vi "Interpret Driver Controls.vi"() -> ()   [LabVIEW 2018]
uses:
  <vilib>/Rock Robotics/WPI/DriverStation/WPI_DriverStationDerivedRobotMode.ctl
  Robot Global Data.vi
  SubSystems/Controllers/Driver Controller/Driver Controller Global.vi
  SubSystems/Drive Train/Drive Train Global.vi
  SubSystems/Lift/Lift Global.vi
  <vilib>/addons/control/pid/pid.llb/PID (DBL).vi
  SubSystems/Controllers/Manipulator Controlller/Manipulator Controller Global.vi
  SubSystems/HAB Climber/HAB Climber Global.vi
  SubSystems/Hatch Panel Intake/Hatch Panel Intake Global.vi
  SubSystems/Cargo Intake/Cargo Intake Global.vi
  <vilib>/addons/control/pid/NI_PID_pid.lvlib
panel:
  in  "Last Move Deadband":u32=500
  in  "Last Time Auto":u32=1171826
  in  "Camera Tracking":T1={"proportional gain (Kc)"=0.06, "integral time (Ti, min)"=0.0, "derivative time (Td, min)"=0.0}
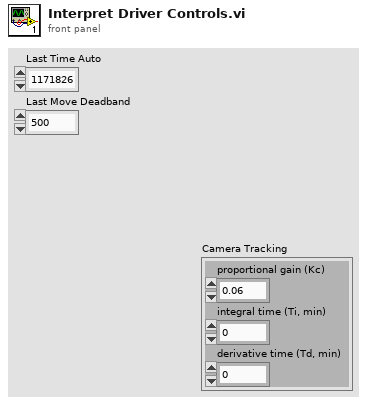
[diagram p1: front panel]
types:
  T1 = cluster{"proportional gain (Kc)":dbl, "integral time (Ti, min)":dbl, "derivative time (Td, min)":dbl}
  T2 = enum16{"Manual", "Hatch Panel Zone 1", "Hatch Panel Zone 2", "Hatch Panel Zone 3", "Cargo Zone 1", "Cargo Zone 2", "Cargo Zone 3", "Cargo Ship Zone"}
  T3 = cluster{"Rollover":dbl, "Yaw":dbl, "Cont Yaw":dbl}
  T4 = typedef "WPI_DriverStationDerivedRobotMode.ctl" = enum16{"Init", "Execute", "Stop"}
  T5 = enum16{"Hatch Panel Zone 1", "Hatch Panel Zone 2", "Hatch Panel Zone 3", "Cargo Zone 1", "Cargo Zone 2", "Cargo Zone 3", "Cargo Ship Zone"}
  T6 = cluster{"offsetAngle H":dbl, "offsetAngle V":dbl, "area":dbl, "skew":dbl, "validTarget":dbl, "latency":dbl}
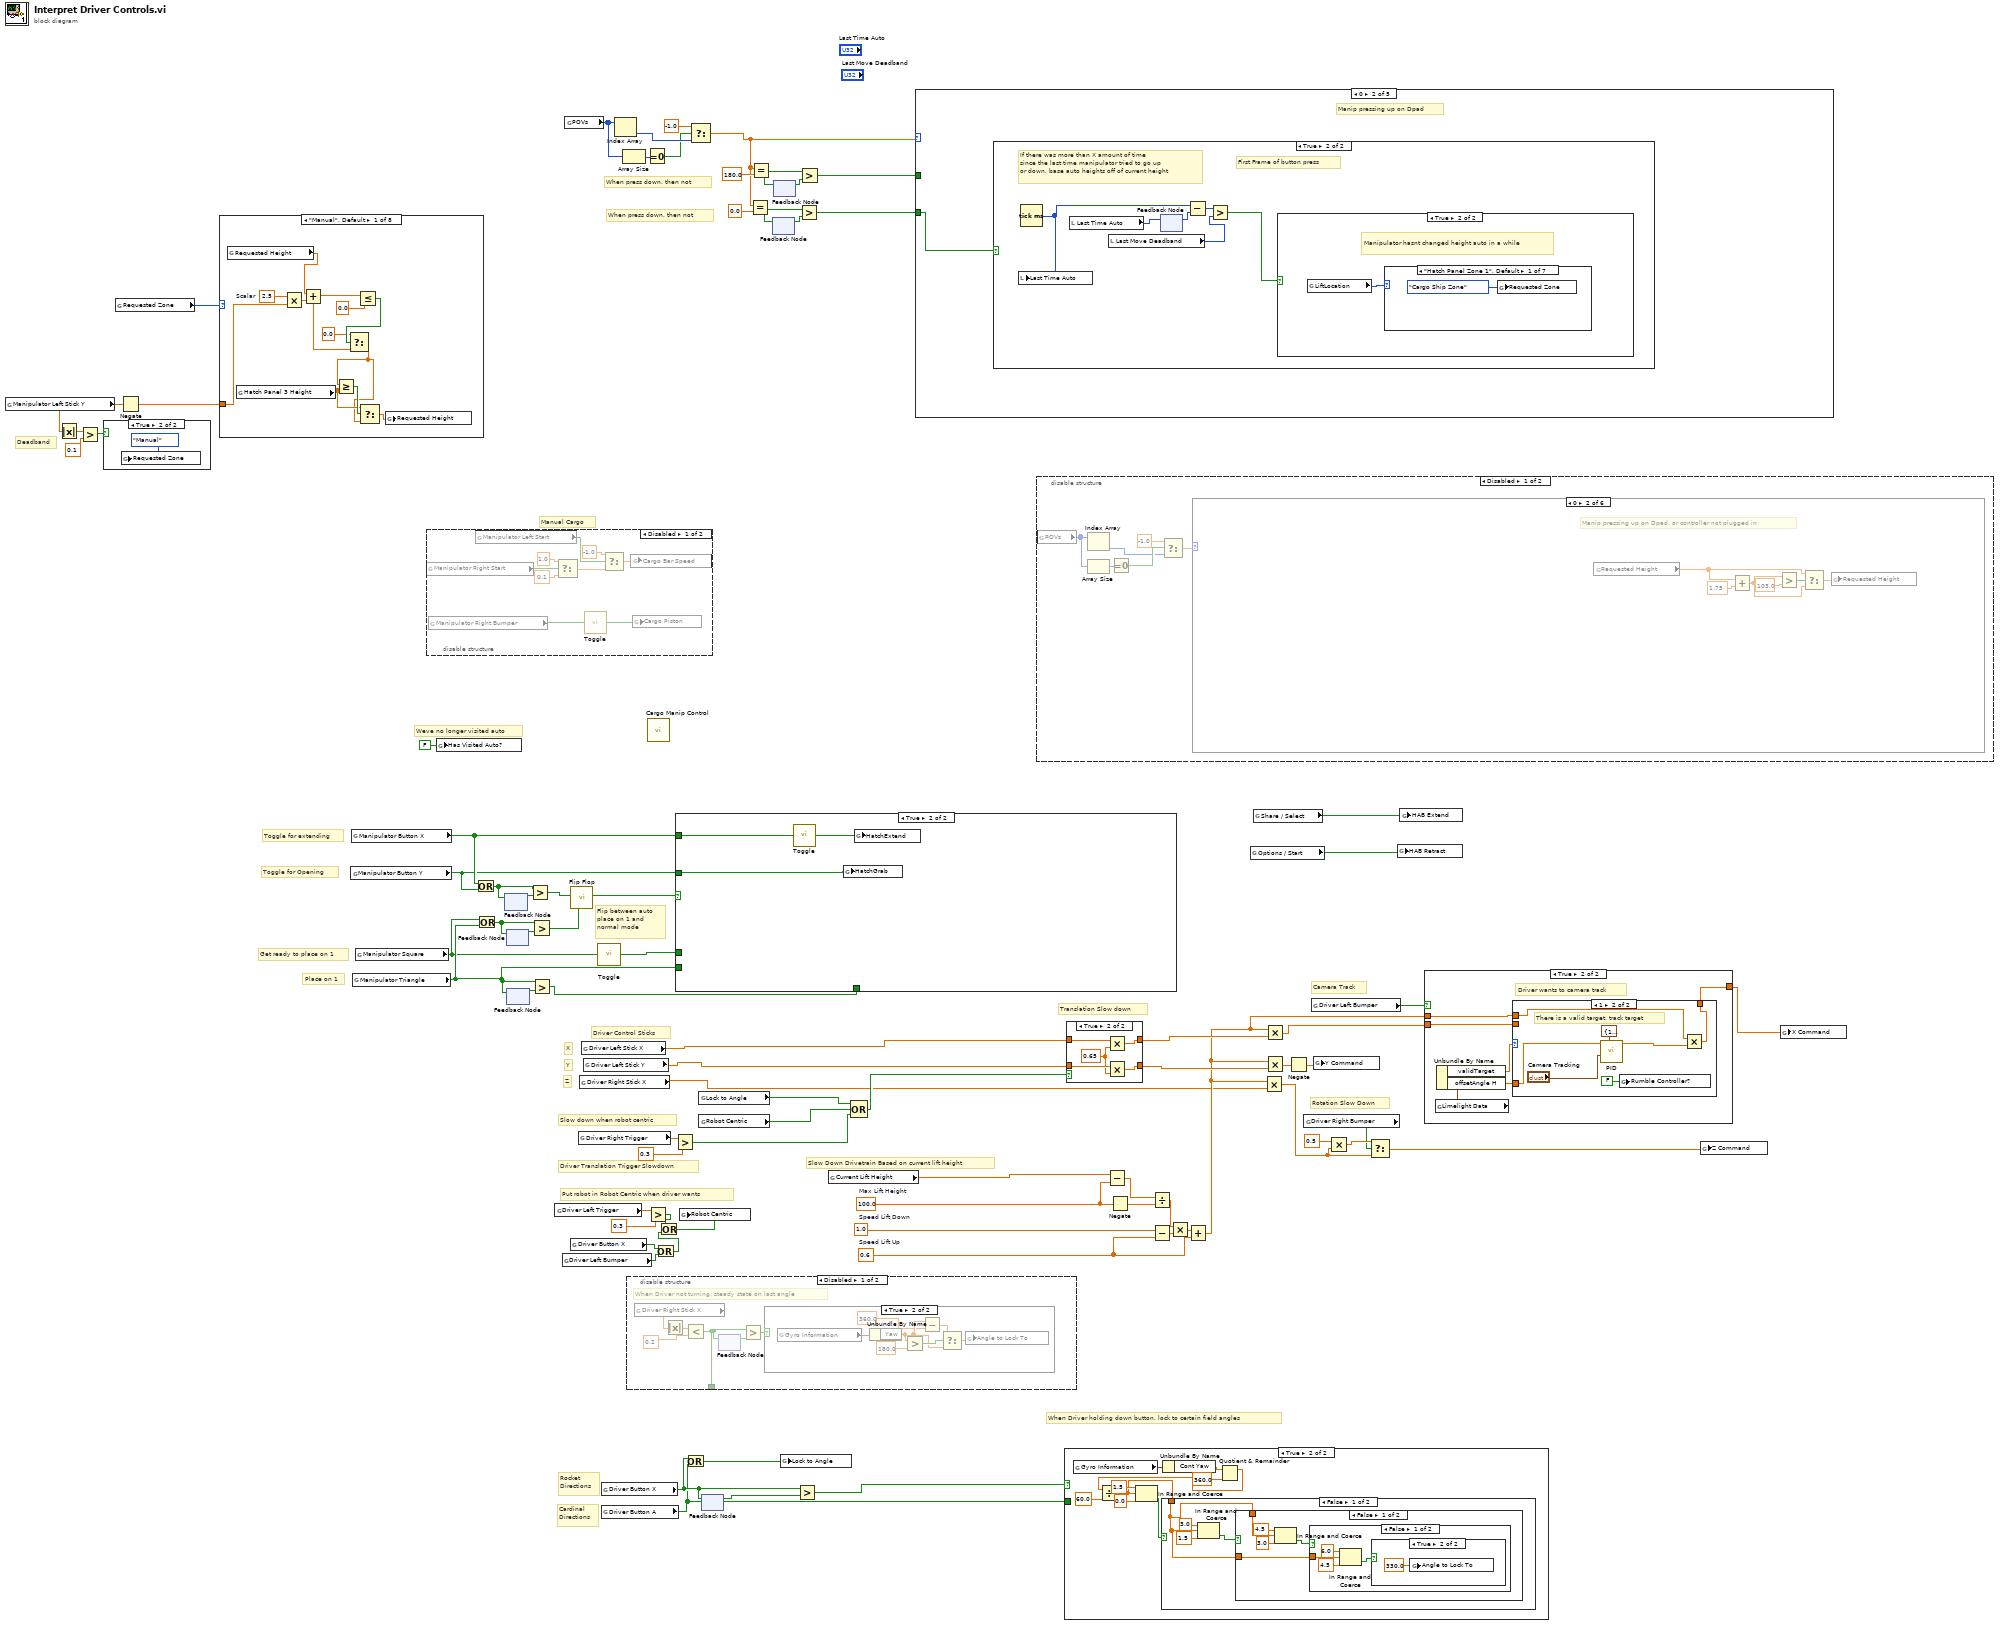
[diagram p0: block diagram]
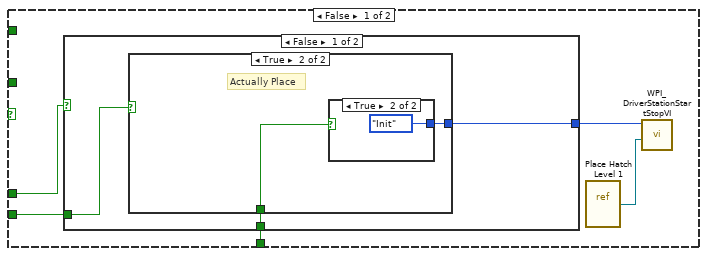
[diagram p2: hidden frame]
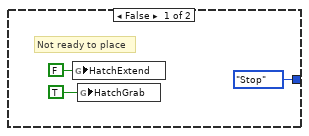
[diagram p3: hidden frame]
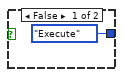
[diagram p4: hidden frame]
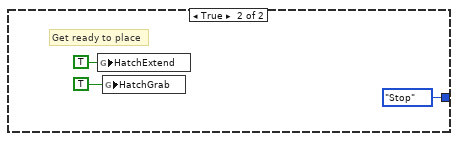
[diagram p5: hidden frame]
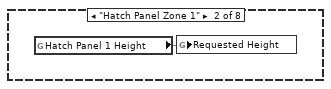
[diagram p7: hidden frame]
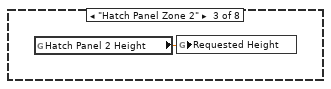
[diagram p8: hidden frame]
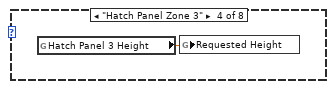
[diagram p9: hidden frame]
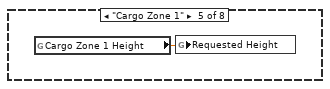
[diagram p10: hidden frame]
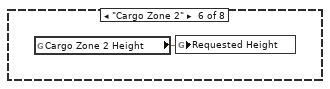
[diagram p11: hidden frame]
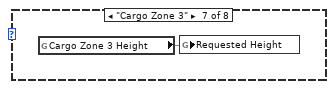
[diagram p12: hidden frame]
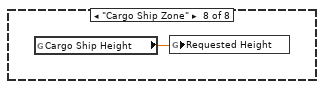
[diagram p13: hidden frame]
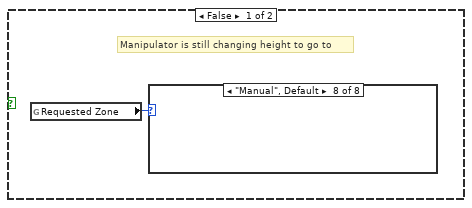
[diagram p16: hidden frame]
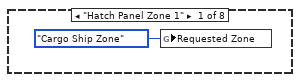
[diagram p17: hidden frame]
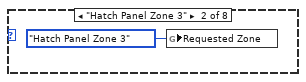
[diagram p18: hidden frame]
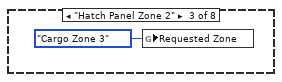
[diagram p19: hidden frame]
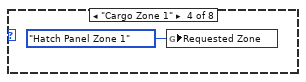
[diagram p20: hidden frame]
diagram:
  w61 = 0.6  # Speed Lift Up
  w65 = 1.0  # Speed Lift Down
  w59 = 100.0  # Max Lift Height
  # "Toggle for Opening"
  # "Toggle for extending"
  # "Place on 1"
  # "Get ready to place on 1"
  # "Flip between auto\nplace on 1 and \nnormal mode"
  # "When press down, then not"
  # "When press down, then not"
  # "Deadband"
  # "Manual Cargo"
  # "Weve no longer visited auto"
  # "Camera Track"
  # "Rotation Slow Down"
  # "Rocket\nDirections"
  # "Cardinal\nDirections"
  # "When Driver holding down button, lock to certain field angles"
  # "Slow Down Drivetrain Based on current lift height"
  # "Put robot in Robot Centric when driver wants"
  # "Slow down when robot centric"
  # "Driver Translation Trigger Slowdown"
  # "Translation Slow down"
  # "Z"
  # "Y"
  # "X"
  # "Driver Control Sticks"
  n1 = global read "Manipulator Controller Global.vi" "Manipulator Left Stick Y"() -> (w30:dbl)
  n2 = Absolute Value(x=w30) -> (abs(x)=w33:dbl)
  n3 = Greater?(x=w33, y=0.1) -> (0:w31:bool)
  n4 = case shown="True" w31 {
    frame False {
    }
    frame True {
      n5 = global write "Lift Global.vi" "Requested Zone"(T2."Manual" ("Requested Zone")) -> ()
    }
  }
  n6 = global read "Lift Global.vi" "Requested Zone"() -> (w34:T2)
  n7 = Negate(x=w30) -> (-x=w29:dbl)
  n8 = case shown="\"Manual\", Default" w34 {
    tunnel: w29 -> [w91 _ _ _ _ _ _ _]
    frame "Manual", Default {
      w90 = 2.5  # Scalar
      n9 = global read "Lift Global.vi" "Requested Height"() -> (w93:dbl)
      n10 = global read "Lift Global.vi" "Hatch Panel 3 Height"() -> (w84:dbl)
      n11 = Multiply(x=w90, y=w91) -> (x*y=w92:dbl)
      n12 = Add(x=w93, y=w92) -> (x+y=w86:dbl)
      n13 = Less Or Equal?(x=w86, y=0.0) -> (x <= y?=w88:bool)
      n14 = Select(t=0.0, s=w88, f=w86) -> (s? t:f=w83:dbl)
      n15 = Greater Or Equal?(x=w83, y=w84) -> (x >= y?=w85:bool)
      n16 = Select(t=w84, s=w85, f=w83) -> (s? t:f=w82:dbl)
      n17 = global write "Lift Global.vi" "Requested Height"(w82) -> ()
    }
    frame "Hatch Panel Zone 1" {
      n18 = global read "Lift Global.vi" "Hatch Panel 1 Height"() -> (w94:dbl)
      n19 = global write "Lift Global.vi" "Requested Height"(w94) -> ()
    }
    frame "Hatch Panel Zone 2" {
      n20 = global read "Lift Global.vi" "Hatch Panel 2 Height"() -> (w95:dbl)
      n21 = global write "Lift Global.vi" "Requested Height"(w95) -> ()
    }
    frame "Hatch Panel Zone 3" {
      n22 = global read "Lift Global.vi" "Hatch Panel 3 Height"() -> (w96:dbl)
      n23 = global write "Lift Global.vi" "Requested Height"(w96) -> ()
    }
    frame "Cargo Zone 1" {
      n24 = global read "Lift Global.vi" "Cargo Zone 1 Height"() -> (w97:dbl)
      n25 = global write "Lift Global.vi" "Requested Height"(w97) -> ()
    }
    frame "Cargo Zone 2" {
      n26 = global read "Lift Global.vi" "Cargo Zone 2 Height"() -> (w98:dbl)
      n27 = global write "Lift Global.vi" "Requested Height"(w98) -> ()
    }
    frame "Cargo Zone 3" {
      n28 = global read "Lift Global.vi" "Cargo Zone 3 Height"() -> (w99:dbl)
      n29 = global write "Lift Global.vi" "Requested Height"(w99) -> ()
    }
    frame "Cargo Ship Zone" {
      n30 = global read "Lift Global.vi" "Cargo Ship Height"() -> (w100:dbl)
      n31 = global write "Lift Global.vi" "Requested Height"(w100) -> ()
    }
  }
  n32 = global read "Manipulator Controller Global.vi" "Manipulator Button Y"() -> (w16:bool)
  n33 = global read "Manipulator Controller Global.vi" "Manipulator Button X"() -> (w17:bool)
  n34 = global read "Manipulator Controller Global.vi" "Manipulator Triangle"() -> (w6:bool)
  n35 = global read "Manipulator Controller Global.vi" "Manipulator Square"() -> (w5:bool)
  n36 = disable-structure shown="Disabled" {
    frame Disabled {
      n37 = global read "Manipulator Controller Global.vi" "Manipulator Right Start"() -> (w106:bool)
      n38 = global read "Manipulator Controller Global.vi" "Manipulator Right Bumper"() -> (w109:bool)
      n39 = global read "Manipulator Controller Global.vi" "Manipulator Left Start"() -> (w105:bool)
      n40 = Select(t=1.0, s=w106, f=0.1) -> (s? t:f=w104:dbl)
      n41 = call "Toggle.vi"("Input"=w109) -> ("Output"=w108:bool)
      n42 = Select(t=-1.0, s=w105, f=w104) -> (s? t:f=w107:dbl)
      n43 = global write "Cargo Intake Global.vi" "Cargo Bar Speed"(w107) -> ()
      n44 = global write "Cargo Intake Global.vi" "Cargo Piston"(w108) -> ()
    }
    frame Enabled {
    }
  }
  n45 = global write "Robot Global Data.vi" "Has Visited Auto?"(FALSE ("Has Visited Auto?")) -> ()
  n46 = Or(x=w17, y=w16) -> (x .or. y?=w14:bool)
  n47 = Or(x=w5, y=w6) -> (x .or. y?=w11:bool)
  n48 = feedback-in #1(w14) -> ()
  n49 = feedback #1() -> (w15:bool)  [unwired: 1 in]
  n50 = feedback #2() -> (w12:bool)  [unwired: 1 in]
  n51 = feedback-in #2(w11) -> ()
  n52 = feedback #3() -> (w8:bool)  [unwired: 1 in]
  n53 = feedback-in #3(w6) -> ()
  n54 = Greater?(x=w14, y=w15) -> (0:w13:bool)
  n55 = Greater?(x=w11, y=w12) -> (0:w10:bool)
  n56 = Greater?(x=w6, y=w8) -> (0:w7:bool)
  n57 = global read "Driver Controller Global.vi" "Driver Left Trigger"() -> (w77:dbl)
  n58 = global read "Driver Controller Global.vi" "Driver Left Bumper"() -> (w44:bool)
  n59 = global read "Manipulator Controller Global.vi" "POVs"() -> (w38:i16[])
  n60 = call "Flip Flop.vi"("Line 2"=w10, "Line 1"=w13) -> ("Switch"=w9:bool)  [unwired: 9 in]
  n61 = global read "Driver Controller Global.vi" "Driver Button X"() -> (w45:bool)
  n62 = global read "Driver Controller Global.vi" "Driver Right Trigger"() -> (w80:dbl)
  n63 = global read "Driver Controller Global.vi" "Driver Right Stick X"() -> (w1:dbl)
  n64 = global read "Driver Controller Global.vi" "Driver Left Stick X"() -> (w3:dbl)
  n65 = global read "Driver Controller Global.vi" "Driver Left Stick Y"() -> (w2:dbl)
  n66 = call "Toggle.vi"("Input"=w5) -> ("Output"=w4:bool)
  n67 = global read "Driver Controller Global.vi" "Driver Button X"() -> (w57:bool)
  n68 = global read "Driver Controller Global.vi" "Driver Button A"() -> (w55:bool)
  n69 = Index Array(array=w38) -> (element=w35:i16)  [unwired: 1 in]
  n70 = Array Size(array=w38) -> (size(s)=w37:i32)
  n71 = disable-structure shown="Disabled" {
    disable-tunnel: [w110 _] -> _
    frame Disabled {
      # "When Driver not turning, steady state on last angle"
      n72 = global read "Driver Controller Global.vi" "Driver Right Stick X"() -> (w111:dbl)
      n73 = Absolute Value(x=w111) -> (abs(x)=w115:dbl)
      n74 = Less?(x=w115, y=0.2) -> (x < y?=w110:bool)
      n75 = feedback #4() -> (w113:bool)  [unwired: 1 in]
      n76 = feedback-in #4(w110) -> ()
      n77 = Greater?(x=w110, y=w113) -> (0:w112:bool)
      n78 = case shown="True" w112 {
        frame False {
        }
        frame True {
          n79 = global read "Drive Train Global.vi" "Gyro Information"() -> (w122:T3)
          n80 = Unbundle By Name(w122) -> ("Yaw"=w119:dbl)
          n81 = Greater?(x=w119, y=180.0) -> (0:w120:bool)
          n82 = Subtract(x=w119, y=360.0) -> (x-y=w117:dbl)
          n83 = Select(t=w117, s=w120, f=w119) -> (s? t:f=w116:dbl)
          n84 = global write "Drive Train Global.vi" "Angle to Lock To"(w116) -> ()
        }
      }
    }
    frame Enabled {
    }
  }
  n85 = Equal To 0?(x=w37) -> (x = 0?=w28:bool)
  n86 = call "Cargo Manip Control.vi"() -> ()  [unwired: 12 in]
  n87 = Greater?(x=w77, y=0.3) -> (0:w53:bool)
  n88 = Or(x=w45, y=w44) -> (x .or. y?=w46:bool)
  n89 = Or(x=w53, y=w46) -> (x .or. y?=w51:bool)
  n90 = Greater?(x=w80, y=0.3) -> (0:w72:bool)
  n91 = case shown="True" w9 {
    tunnel: w16 -> [_ w141]
    tunnel: w17 -> [_ w142]
    tunnel: w4 -> [w127 _]
    tunnel: w7 -> [w124 _]
    tunnel: w6 -> [w123 _]
    frame False {
      n92 = case shown="False" w127 {
        tunnel: [w130 WPI_DriverStationDerivedRobotMode."Stop" ("Call Context")] -> w125
        tunnel: w124 -> [w129 _]
        tunnel: w123 -> [w128 _]
        frame False {
          n93 = case shown="True" w128 {
            tunnel: [WPI_DriverStationDerivedRobotMode."Stop" ("Call Context") w135] -> w130
            tunnel: w129 -> [_ w134]
            frame False {
              # "Not ready to place"
              n94 = global write "Hatch Panel Intake Global.vi" "HatchExtend"(FALSE ("HatchExtend")) -> ()
              n95 = global write "Hatch Panel Intake Global.vi" "HatchGrab"(TRUE ("HatchExtend")) -> ()
            }
            frame True {
              # "Actually Place"
              n96 = case shown="True" w134 {
                tunnel: [WPI_DriverStationDerivedRobotMode."Execute" ("Call Context") WPI_DriverStationDerivedRobotMode."Init" ("Call Context")] -> w135
                frame False {
                }
                frame True {
                }
              }
            }
          }
        }
        frame True {
          # "Get ready to place"
          n97 = global write "Hatch Panel Intake Global.vi" "HatchExtend"(TRUE ("HatchExtend")) -> ()
          n98 = global write "Hatch Panel Intake Global.vi" "HatchGrab"(TRUE ("HatchExtend")) -> ()
        }
      }
      n99 = vi-ref "Place Hatch Level 1.vi"() -> (w126:refnum<vi>)
      n100 = call <vilib>:"WPI_DriverStationStartStopVI.vi"("VI in"=w126, "Call Context"=w125) -> ()  [unwired: 10 in]
    }
    frame True {
      n101 = call "Toggle.vi"("Input"=w142) -> ("Output"=w143:bool)
      n102 = global write "Hatch Panel Intake Global.vi" "HatchGrab"(w141) -> ()
      n103 = global write "Hatch Panel Intake Global.vi" "HatchExtend"(w143) -> ()
    }
  }
  n104 = global write "Drive Train Global.vi" "Robot Centric"(w51) -> ()
  n105 = Or(x=w57, y=w55) -> (x .or. y?=w54:bool)
  n106 = Select(t=-1.0, s=w28, f=w35) -> (s? t:f=w20:dbl)
  n107 = global read "Drive Train Global.vi" "Lock to Angle"() -> (w52:bool)
  n108 = global read "Drive Train Global.vi" "Robot Centric"() -> (w71:bool)
  n109 = feedback #5() -> (w58:bool)  [unwired: 1 in]
  n110 = feedback-in #5(w57) -> ()
  n111 = Equal?(x=w20, y=0.0) -> (x = y?=w23:bool)
  n112 = Equal?(x=w20, y=180.0) -> (x = y?=w25:bool)
  n113 = feedback #6() -> (w22:bool)  [unwired: 1 in]
  n114 = feedback-in #6(w23) -> ()
  n115 = feedback-in #7(w25) -> ()
  n116 = feedback #7() -> (w26:bool)  [unwired: 1 in]
  n117 = global write "Drive Train Global.vi" "Lock to Angle"(w54) -> ()
  n118 = Greater?(x=w57, y=w58) -> (0:w56:bool)
  n119 = Greater?(x=w23, y=w22) -> (0:w19:bool)
  n120 = Greater?(x=w25, y=w26) -> (0:w24:bool)
  n121 = global read "Lift Global.vi" "Current Lift Height"() -> (w67:dbl)
  n122 = Compound Arithmetic op=OR(w52, w71, w72) -> (w70:bool)
  n123 = case shown="0" w20 {
    tunnel: w24 -> [_ _ w167 _ _]
    tunnel: w19 -> [_ w144 _ _ _]
    frame -1, Default {
      # "Nothing on the D-Pad is pressed!"
    }
    frame 0 {
      # "Manip pressing up on Dpad"
      n124 = case shown="True" w144 {
        frame False {
          # "Still pressing button, do nothing"
        }
        frame True {
          # "First Frame of button press"
          # "If there was more than X amount of time\nsince the last time manipulator tried to go up\nor down, base auto heights off of current height"
          n125 = Tick Count (ms)() -> (millisecond timer value=w147:u32)
          n126 = local write "Last Time Auto"(w147) -> ()
          n127 = local read "Last Time Auto"() -> (w146:u32)
          n128 = local read "Last Move Deadband"() -> (w148:u32)
          n129 = feedback #8() -> (w145:u32)  [unwired: 1 in]
          n130 = feedback-in #8(w146) -> ()
          n131 = Subtract(x=w147, y=w145) -> (x-y=w150:u32)
          n132 = Greater?(x=w150, y=w148) -> (0:w149:bool)
          n133 = case shown="True" w149 {
            frame False {
              # "Manipulator is still changing height to go to"
              n134 = global read "Lift Global.vi" "Requested Zone"() -> (w151:T2)
              n135 = case shown="\"Manual\", Default" w151 {
                frame "Hatch Panel Zone 1" {
                  n136 = global write "Lift Global.vi" "Requested Zone"(T2."Cargo Ship Zone" ("Requested Zone")) -> ()
                }
                frame "Hatch Panel Zone 3" {
                  n137 = global write "Lift Global.vi" "Requested Zone"(T2."Hatch Panel Zone 3" ("Requested Zone")) -> ()
                }
                frame "Hatch Panel Zone 2" {
                  n138 = global write "Lift Global.vi" "Requested Zone"(T2."Cargo Zone 3" ("Requested Zone")) -> ()
                }
                frame "Cargo Zone 1" {
                  n139 = global write "Lift Global.vi" "Requested Zone"(T2."Hatch Panel Zone 1" ("Requested Zone")) -> ()
                }
                frame "Cargo Zone 2" {
                  n140 = global write "Lift Global.vi" "Requested Zone"(T2."Hatch Panel Zone 2" ("Requested Zone")) -> ()
                }
                frame "Cargo Zone 3" {
                  n141 = global write "Lift Global.vi" "Requested Zone"(T2."Hatch Panel Zone 3" ("Requested Zone")) -> ()
                }
                frame "Cargo Ship Zone" {
                  n142 = global write "Lift Global.vi" "Requested Zone"(T2."Cargo Zone 2" ("Requested Zone")) -> ()
                }
                frame "Manual", Default {
                }
              }
            }
            frame True {
              # "Manipulator hasnt changed height auto in a while"
              n143 = global read "Lift Global.vi" "LiftLocation"() -> (w159:T5)
              n144 = case shown="\"Hatch Panel Zone 1\", Default" w159 {
                frame "Hatch Panel Zone 1", Default {
                  n145 = global write "Lift Global.vi" "Requested Zone"(T2."Cargo Ship Zone" ("Requested Zone")) -> ()
                }
                frame "Hatch Panel Zone 3" {
                  n146 = global write "Lift Global.vi" "Requested Zone"(T2."Hatch Panel Zone 3" ("Requested Zone")) -> ()
                }
                frame "Hatch Panel Zone 2" {
                  n147 = global write "Lift Global.vi" "Requested Zone"(T2."Cargo Zone 3" ("Requested Zone")) -> ()
                }
                frame "Cargo Zone 1" {
                  n148 = global write "Lift Global.vi" "Requested Zone"(T2."Hatch Panel Zone 1" ("Requested Zone")) -> ()
                }
                frame "Cargo Zone 2" {
                  n149 = global write "Lift Global.vi" "Requested Zone"(T2."Hatch Panel Zone 2" ("Requested Zone")) -> ()
                }
                frame "Cargo Zone 3" {
                  n150 = global write "Lift Global.vi" "Requested Zone"(T2."Hatch Panel Zone 3" ("Requested Zone")) -> ()
                }
                frame "Cargo Ship Zone" {
                  n151 = global write "Lift Global.vi" "Requested Zone"(T2."Cargo Zone 2" ("Requested Zone")) -> ()
                }
              }
            }
          }
        }
      }
    }
    frame 180 {
      # "Manip pressing down on Dpad"
      n152 = case shown="True" w167 {
        frame False {
          # "Still pressing button, do nothing"
        }
        frame True {
          # "First frame of button press"
          # "If there was more than X amount of time\nsince the last time manipulator tried to go up\nor down, base auto heights off of current height"
          n153 = Tick Count (ms)() -> (millisecond timer value=w172:u32)
          n154 = local write "Last Time Auto"(w172) -> ()
          n155 = local read "Last Time Auto"() -> (w169:u32)
          n156 = local read "Last Move Deadband"() -> (w171:u32)
          n157 = feedback #9() -> (w168:u32)  [unwired: 1 in]
          n158 = feedback-in #9(w169) -> ()
          n159 = Subtract(x=w172, y=w168) -> (x-y=w173:u32)
          n160 = Greater?(x=w173, y=w171) -> (0:w170:bool)
          n161 = case shown="False" w170 {
            frame False {
              # "Manipulator is still changing height to go to"
              n162 = global read "Lift Global.vi" "Requested Zone"() -> (w174:T2)
              n163 = case shown="\"Cargo Ship Zone\"" w174 {
                frame "Hatch Panel Zone 1" {
                  n164 = global write "Lift Global.vi" "Requested Zone"(T2."Cargo Zone 1" ("Requested Zone")) -> ()
                }
                frame "Hatch Panel Zone 3" {
                  n165 = global write "Lift Global.vi" "Requested Zone"(T2."Cargo Zone 3" ("Requested Zone")) -> ()
                }
                frame "Hatch Panel Zone 2" {
                  n166 = global write "Lift Global.vi" "Requested Zone"(T2."Cargo Zone 2" ("Requested Zone")) -> ()
                }
                frame "Cargo Zone 1" {
                  n167 = global write "Lift Global.vi" "Requested Zone"(T2."Cargo Zone 1" ("Requested Zone")) -> ()
                }
                frame "Cargo Zone 2" {
                  n168 = global write "Lift Global.vi" "Requested Zone"(T2."Cargo Ship Zone" ("Requested Zone")) -> ()
                }
                frame "Cargo Zone 3" {
                  n169 = global write "Lift Global.vi" "Requested Zone"(T2."Hatch Panel Zone 2" ("Requested Zone")) -> ()
                }
                frame "Cargo Ship Zone" {
                  n170 = global write "Lift Global.vi" "Requested Zone"(T2."Hatch Panel Zone 1" ("Requested Zone")) -> ()
                }
                frame "Manual", Default {
                }
              }
            }
            frame True {
              # "Manipulator hasnt changed height auto in a while"
              n171 = global read "Lift Global.vi" "LiftLocation"() -> (w182:T5)
              n172 = case shown="\"Hatch Panel Zone 1\", Default" w182 {
                frame "Hatch Panel Zone 1", Default {
                  n173 = global write "Lift Global.vi" "Requested Zone"(T2."Cargo Zone 1" ("Requested Zone")) -> ()
                }
                frame "Hatch Panel Zone 3" {
                  n174 = global write "Lift Global.vi" "Requested Zone"(T2."Cargo Zone 3" ("Requested Zone")) -> ()
                }
                frame "Hatch Panel Zone 2" {
                  n175 = global write "Lift Global.vi" "Requested Zone"(T2."Cargo Zone 2" ("Requested Zone")) -> ()
                }
                frame "Cargo Zone 1" {
                  n176 = global write "Lift Global.vi" "Requested Zone"(T2."Cargo Zone 1" ("Requested Zone")) -> ()
                }
                frame "Cargo Zone 2" {
                  n177 = global write "Lift Global.vi" "Requested Zone"(T2."Cargo Ship Zone" ("Requested Zone")) -> ()
                }
                frame "Cargo Zone 3" {
                  n178 = global write "Lift Global.vi" "Requested Zone"(T2."Hatch Panel Zone 2" ("Requested Zone")) -> ()
                }
                frame "Cargo Ship Zone" {
                  n179 = global write "Lift Global.vi" "Requested Zone"(T2."Hatch Panel Zone 1" ("Requested Zone")) -> ()
                }
              }
            }
          }
        }
      }
    }
    frame 90 {
      # "Go to Cargo in Cargo Ship Height"
      # "Right on D-Pad"
      n180 = global write "Lift Global.vi" "Requested Zone"(T2."Cargo Ship Zone" ("Requested Zone")) -> ()
    }
    frame 270 {
      # "Go to Hatch Level 1 Height"
      # "Left on D-Pad"
      n181 = global write "Lift Global.vi" "Requested Zone"(T2."Hatch Panel Zone 1" ("Requested Zone")) -> ()
    }
  }
  n182 = disable-structure shown="Disabled" {
    frame Disabled {
      n183 = global read "Manipulator Controller Global.vi" "POVs"() -> (w197:i16[])
      n184 = Index Array(array=w197) -> (element=w192:i16)  [unwired: 1 in]
      n185 = Array Size(array=w197) -> (size(s)=w196:i32)
      n186 = Equal To 0?(x=w196) -> (x = 0?=w194:bool)
      n187 = Select(t=-1.0, s=w194, f=w192) -> (s? t:f=w195:dbl)
      n188 = case shown="0" w195 {
        frame -1 {
          # "If the value changed (manip pressed button)\nchange set lift height to match"
          # "When button goes from\nnot pressed to pressed"
          n189 = global read "Manipulator Controller Global.vi" "Manipulator Square"() -> (w203:bool)
          n190 = feedback #10() -> (w204:bool)  [unwired: 1 in]
          n191 = feedback-in #10(w203) -> ()
          n192 = Greater?(x=w203, y=w204) -> (0:w200:bool)
          n193 = feedback #11() -> (w198:dbl)  [unwired: 1 in]
          n194 = feedback #12() -> (w202:dbl)  [unwired: 1 in]
          n195 = case shown="False" w200 {
            tunnel: [w214 w229] -> w199
            tunnel: w202 -> [w215 w228]
            frame False {
              # "When button goes from\nnot pressed to pressed"
              n196 = global read "Manipulator Controller Global.vi" "Manipulator Triangle"() -> (w217:bool)
              n197 = feedback #13() -> (w216:bool)  [unwired: 1 in]
              n198 = feedback-in #13(w217) -> ()
              n199 = Greater?(x=w217, y=w216) -> (0:w213:bool)
              n200 = case shown="True" w213 {
                tunnel: w215 -> [w218 w220]
                tunnel: [w218 w222] -> w214
                frame False {
                }
                frame True {
                  # "If counter smaller than 5\nadd 1"
                  n201 = Less?(x=w220, y=5.0) -> (x < y?=w219:bool)
                  n202 = case shown="True" w219 {
                    tunnel: [w223 w225] -> w222
                    tunnel: w220 -> [w223 w224]
                    frame False {
                    }
                    frame True {
                      n203 = Increment(x=w224) -> (x+1=w225:dbl)
                    }
                  }
                }
              }
            }
            frame True {
              # "If counter bigger than 0\nsubtract 1"
              n204 = Greater?(x=w228, y=0.0) -> (0:w227:bool)
              n205 = case shown="False" w227 {
                tunnel: [0.0 ("y") w232] -> w229
                tunnel: w228 -> [_ w231]
                frame False {
                }
                frame True {
                  n206 = Decrement(x=w231) -> (x-1=w232:dbl)
                }
              }
            }
          }
          n207 = feedback-in #11(w199) -> ()
          n208 = Not Equal?(x=w199, y=w198) -> (x != y?=w201:bool)
          n209 = case shown="True" w201 {
            tunnel: w199 -> [_ w205]
            frame False {
              # "Manipulator didnt request change"
            }
            frame True {
              # "Set height request to new value"
              n210 = case shown="0, Default" w205 {
                tunnel: [w207 w208 w209 w210 w211 w212] -> w206
                frame 0, Default {
                  n211 = global read "Lift Global.vi" "Cargo Zone 1 Height"() -> (w207:dbl)
                }
                frame 1 {
                  n212 = global read "Lift Global.vi" "Hatch Panel 1 Height"() -> (w208:dbl)
                }
                frame 2 {
                  n213 = global read "Lift Global.vi" "Cargo Zone 2 Height"() -> (w209:dbl)
                }
                frame 3 {
                  n214 = global read "Lift Global.vi" "Hatch Panel 2 Height"() -> (w210:dbl)
                }
                frame 4 {
                  n215 = global read "Lift Global.vi" "Cargo Zone 3 Height"() -> (w211:dbl)
                }
                frame 5 {
                  n216 = global read "Lift Global.vi" "Hatch Panel 3 Height"() -> (w212:dbl)
                }
              }
              n217 = global write "Lift Global.vi" "Requested Height"(w206) -> ()
            }
          }
          n218 = global write "Lift Global.vi" "Lift Auto Position"(w199) -> ()
          n219 = feedback-in #12(w199) -> ()
        }
        frame 0 {
          # "Manip pressing up on Dpad, or controller not plugged in"
          n220 = global read "Lift Global.vi" "Requested Height"() -> (w234:dbl)
          n221 = Add(x=w234, y=1.75) -> (x+y=w233:dbl)
          n222 = Greater?(x=w233, y=103.0) -> (0:w235:bool)
          n223 = Select(t=w234, s=w235, f=w233) -> (s? t:f=w236:dbl)
          n224 = global write "Lift Global.vi" "Requested Height"(w236) -> ()
        }
        frame 180 {
          # "Manip pressing down on Dpad"
          n225 = global read "Lift Global.vi" "Requested Height"() -> (w239:dbl)
          n226 = Add(x=w239, y=-1.0) -> (x+y=w241:dbl)
          n227 = Less?(x=w241, y=0.0) -> (x < y?=w242:bool)
          n228 = Select(t=w239, s=w242, f=w241) -> (s? t:f=w240:dbl)
          n229 = global write "Lift Global.vi" "Requested Height"(w240) -> ()
        }
        frame 90 {
          # "Go to Cargo in Cargo Ship Height"
          # "Right on D-Pad"
          n230 = global read "Lift Global.vi" "Cargo Ship Height"() -> (w245:dbl)
          n231 = global write "Lift Global.vi" "Requested Height"(w245) -> ()
        }
        frame 270 {
          # "Go to Hatch Level 1 Height"
          # "Left on D-Pad"
          n232 = global read "Lift Global.vi" "Hatch Panel 1 Height"() -> (w246:dbl)
          n233 = global write "Lift Global.vi" "Requested Height"(w246) -> ()
        }
        frame -100, Default {
        }
      }
    }
    frame Enabled {
    }
  }
  n234 = case shown="True" w56 {
    tunnel: w55 -> [w248 _]
    frame False {
      n235 = feedback #14() -> (w249:bool)  [unwired: 1 in]
      n236 = feedback-in #14(w248) -> ()
      n237 = Greater?(x=w248, y=w249) -> (0:w247:bool)
      n238 = case shown="True" w247 {
        frame False {
        }
        frame True {
          n239 = global read "Drive Train Global.vi" "Gyro Information"() -> (w256:T3)
          n240 = Unbundle By Name(w256) -> ("Yaw"=w253:dbl)
          n241 = Add(x=w253, y=180.0) -> (x+y=w252:dbl)
          n242 = Divide(x=w252, y=90.0) -> (x/y=w254:dbl)
          n243 = Round To Nearest(number=w254) -> (nearest integer value=w250:dbl)
          n244 = case shown="1" w250 {
            frame 0, Default {
              n245 = global write "Drive Train Global.vi" "Angle to Lock To"(180.0 ("Angle to Lock To")) -> ()
            }
            frame 1 {
              n246 = global write "Drive Train Global.vi" "Angle to Lock To"(270.0 ("Angle to Lock To")) -> ()
            }
            frame 2 {
              n247 = global write "Drive Train Global.vi" "Angle to Lock To"(0.0 ("Angle to Lock To")) -> ()
            }
            frame 3 {
              n248 = global write "Drive Train Global.vi" "Angle to Lock To"(90.0 ("Angle to Lock To")) -> ()
            }
            frame 4 {
              n249 = global write "Drive Train Global.vi" "Angle to Lock To"(180.0 ("Angle to Lock To")) -> ()
            }
          }
        }
      }
    }
    frame True {
      n250 = global read "Drive Train Global.vi" "Gyro Information"() -> (w270:T3)
      n251 = Unbundle By Name(w270) -> ("Cont Yaw"=w268:dbl)
      n252 = Quotient & Remainder(x=w268, y=360.0) -> (x-y*floor(x/y)=w266:dbl)  [unwired: 1 out]
      n253 = Divide(x=w266, y=60.0) -> (x/y=w262:dbl)
      n254 = In Range and Coerce(upper limit=1.5, x=w262, lower limit=0.0) -> (In Range?=w263:bool)  [unwired: 1 out]
      n255 = case shown="False" w263 {
        tunnel: w262 -> [w271 _]
        frame False {
          n256 = In Range and Coerce(upper limit=3.0, x=w271, lower limit=1.5) -> (In Range?=w272:bool)  [unwired: 1 out]
          n257 = case shown="False" w272 {
            tunnel: w271 -> [w277 _]
            tunnel: w271 -> [w275 _]
            frame False {
              n258 = In Range and Coerce(upper limit=4.5, x=w277, lower limit=3.0) -> (In Range?=w276:bool)  [unwired: 1 out]
              n259 = case shown="False" w276 {
                tunnel: w275 -> [w281 _]
                frame False {
                  n260 = In Range and Coerce(upper limit=6.0, x=w281, lower limit=4.5) -> (In Range?=w280:bool)  [unwired: 1 out]
                  n261 = case shown="True" w280 {
                    frame False {
                    }
                    frame True {
                      n262 = global write "Drive Train Global.vi" "Angle to Lock To"(330.0 ("Angle to Lock To")) -> ()
                    }
                  }
                }
                frame True {
                  n263 = global write "Drive Train Global.vi" "Angle to Lock To"(210.0 ("Angle to Lock To")) -> ()
                }
              }
            }
            frame True {
              n264 = global write "Drive Train Global.vi" "Angle to Lock To"(150.0 ("Angle to Lock To")) -> ()
            }
          }
        }
        frame True {
          n265 = global write "Drive Train Global.vi" "Angle to Lock To"(30.0 ("Angle to Lock To")) -> ()
        }
      }
    }
  }
  n266 = case shown="True" w70 {
    tunnel: w2 -> [w289 w294]
    tunnel: [w289 w293] -> w69
    tunnel: [w288 w292] -> w68
    tunnel: w3 -> [w288 w291]
    frame False {
    }
    frame True {
      w290 = 0.65 ("Y Slower")
      n267 = Multiply(x=w291, y=w290) -> (x*y=w292:dbl)
      n268 = Multiply(x=w294, y=w290) -> (x*y=w293:dbl)
    }
  }
  n269 = Subtract(x=w67, y=w59) -> (x-y=w66:dbl)
  n270 = Negate(x=w59) -> (-x=w60:dbl)
  n271 = Divide(x=w66, y=w60) -> (x/y=w64:dbl)
  n272 = Subtract(x=w65, y=w61) -> (x-y=w63:dbl)
  n273 = Multiply(x=w64, y=w63) -> (x*y=w62:dbl)
  n274 = Add(x=w62, y=w61) -> (x+y=w18:dbl)
  n275 = global read "Manipulator Controller Global.vi" "Options / Start"() -> (w42:bool)
  n276 = global read "Manipulator Controller Global.vi" "Share / Select"() -> (w43:bool)
  n277 = Multiply(x=w18, y=w1) -> (x*y=w76:dbl)
  n278 = Multiply(x=w18, y=w68) -> (x*y=w48:dbl)
  n279 = Multiply(x=w18, y=w69) -> (x*y=w41:dbl)
  n280 = Negate(x=w41) -> (-x=w40:dbl)
  n281 = global read "Driver Controller Global.vi" "Driver Right Bumper"() -> (w73:bool)
  n282 = global read "Driver Controller Global.vi" "Driver Left Bumper"() -> (w50:bool)
  n283 = global write "Drive Train Global.vi" "Y Command"(w40) -> ()
  n284 = Multiply(x=0.5, y=w76) -> (x*y=w75:dbl)
  n285 = Select(t=w75, s=w73, f=w76) -> (s? t:f=w49:dbl)
  n286 = global write "HAB Climber Global.vi" "HAB Retract"(w42) -> ()
  n287 = global write "HAB Climber Global.vi" "HAB Extend"(w43) -> ()
  n288 = case shown="True" w50 {
    tunnel: w48 -> [w296 w300]
    tunnel: [w296 w298] -> w47
    tunnel: w18 -> [_ w297]
    frame False {
      # "Driver not attepting to camera track, be normal"
      n289 = global write "Driver Controller Global.vi" "Rumble Controller?"(FALSE ("Rumble Controller?")) -> ()
    }
    frame True {
      # "Driver wants to camera track"
      n290 = global read "Robot Global Data.vi" "Limelight Data"() -> (w302:T6)
      n291 = Unbundle By Name(w302) -> ("validTarget"=w301:dbl, "offsetAngle H"=w299:dbl)
      n292 = case shown="1" w301 {
        tunnel: w300 -> [w303 _]
        tunnel: w299 -> [_ w308]
        tunnel: [w303 w307] -> w298
        tunnel: w297 -> [_ w305]
        frame 0, Default {
          # "No Valid Target, keep using driver controls\nand rumble controller so knows not tracking"
          n293 = global write "Driver Controller Global.vi" "Rumble Controller?"(TRUE ("Rumble Controller?")) -> ()
        }
        frame 1 {
          # "There is a valid target, track target"
          n294 = call-poly <vilib>:"PID.vi"("output range"=cluster{"output high":dbl, "output low":dbl} {"output high"=1.0, "output low"=-1.0}, "PID gains"="Camera Tracking", "setpoint"=w308) -> ("output"=w306:dbl)  [unwired: 7 in, 1 out]
          n295 = global write "Driver Controller Global.vi" "Rumble Controller?"(FALSE ("Rumble Controller?")) -> ()
          n296 = Multiply(x=w305, y=w306) -> (x*y=w307:dbl)
        }
      }
    }
  }
  n297 = global write "Drive Train Global.vi" "Z Command"(w49) -> ()
  n298 = global write "Drive Train Global.vi" "X Command"(w47) -> ()
